vi "turn.vi"   [LabVIEW 2012, in "sumobot 18.lvrbt"]
uses:
  sumobot 18.lvrbt
  <vilib>/NXT/Block Support/NXT_OutputPort.ctl
  <vilib>/NXT/Dual Mode Library/Waits/Wait_Num.vi
  <vilib>/NXT/NXTIO Xnodes/NXTIONodeSubVIs/NXTMoveMotors.vi
  <vilib>/NXT/NXTIO Xnodes/NXTIONodeSubVIs/LEGOStopAllMotors.vi
  <vilib>/NXT/Subs/LVHSConnector.ctl
  <vilib>/NXT/NXTIO Xnodes/AddressXNode/NXTIOAddress.xnode
  <vilib>/NXT/NXTIO Xnodes/NXTIOXNode/NXTIO.xnode
  <vilib>/NXT/LegoClasses/BrickReference/BrickReference.lvclass
types:
  T1 = typedef "NXT_OutputPort.ctl" = u8
  T2 = typedef "LVHSConnector.ctl" = refnum<class "BrickReference.lvclass">
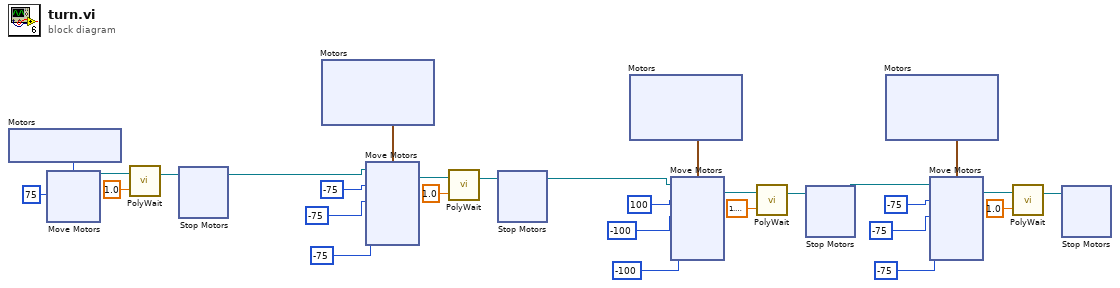
[diagram p0: block diagram]
diagram:
  n1 = xnode "Motors"() -> ("Motor"=w29:T1)
  n2 = xnode "Move Motors"("Power/Speed 1"=i8 75, "Motors"=w29) -> ("NXT/EV3"=w27:T2)  [unwired: 1 in]
  n3 = call-poly <vilib>:"PolyWait.vi"("Time (1 sec)"=sgl 1.0, "NXT/EV3"=w27) -> ("NXT/EV3"=w25:T2)  [unwired: 2 in]
  n4 = xnode "Stop Motors"("NXT/EV3"=w25) -> ("NXT/EV3"=w1:T2)  [unwired: 1 in]
  n5 = xnode "Motors"() -> ("Motor"=w9:cluster{"Port":T1, "Port":T1, "Port":T1})
  n6 = xnode "Move Motors"("Power/Speed 3"=i8 -75 ("Power/Speed 2"), "Power/Speed 2"=i8 -75, "Power/Speed 1"=i8 -75, "Motors"=w9, "NXT/EV3"=w1) -> ("NXT/EV3"=w8:T2)
  n7 = call-poly <vilib>:"PolyWait.vi"("Time (1 sec)"=sgl 1.0, "NXT/EV3"=w8) -> ("NXT/EV3"=w6:T2)  [unwired: 2 in]
  n8 = xnode "Stop Motors"("NXT/EV3"=w6) -> ("NXT/EV3"=w2:T2)  [unwired: 1 in]
  n9 = xnode "Motors"() -> ("Motor"=w24:cluster{"Port":T1, "Port":T1, "Port":T1})
  n10 = xnode "Move Motors"("Power/Speed 3"=i8 -100 ("Power/Speed 2"), "Power/Speed 2"=i8 -100, "Power/Speed 1"=i8 100, "Motors"=w24, "NXT/EV3"=w2) -> ("NXT/EV3"=w23:T2)
  n11 = call-poly <vilib>:"PolyWait.vi"("Time (1 sec)"=sgl 1.4, "NXT/EV3"=w23) -> ("NXT/EV3"=w21:T2)  [unwired: 2 in]
  n12 = xnode "Stop Motors"("NXT/EV3"=w21) -> ("NXT/EV3"=w10:T2)  [unwired: 1 in]
  n13 = xnode "Motors"() -> ("Motor"=w17:cluster{"Port":T1, "Port":T1, "Port":T1})
  n14 = xnode "Move Motors"("Power/Speed 3"=i8 -75 ("Power/Speed 2"), "Power/Speed 2"=i8 -75, "Power/Speed 1"=i8 -75, "Motors"=w17, "NXT/EV3"=w10) -> ("NXT/EV3"=w16:T2)
  n15 = call-poly <vilib>:"PolyWait.vi"("Time (1 sec)"=sgl 1.0, "NXT/EV3"=w16) -> ("NXT/EV3"=w14:T2)  [unwired: 2 in]
  n16 = xnode "Stop Motors"("NXT/EV3"=w14) -> ()  [unwired: 1 in, 1 out]
